vi "WriteToMeasArray.vi"(8 "error in (no error)":errorcluster, 10 "RoomAlert Device Reference":refnum<vi>, 11 "RoomAlert in":refnum<class "RoomAlert.lvclass">) -> (0 "error out":errorcluster, 3 "RoomAlert out":refnum<class "RoomAlert.lvclass">)   [LabVIEW 2018, in "SensorPlugins.lvlib" / "RoomAlert.lvclass"]
doc: "Updates to the measurement array all the values a user may measure from the RoomAlert."
uses:
  RoomAlert.lvclass
  TypeDefinitions/RoomAlertControls.ctl
panel:
  in  "Text Ring":u16(ring)
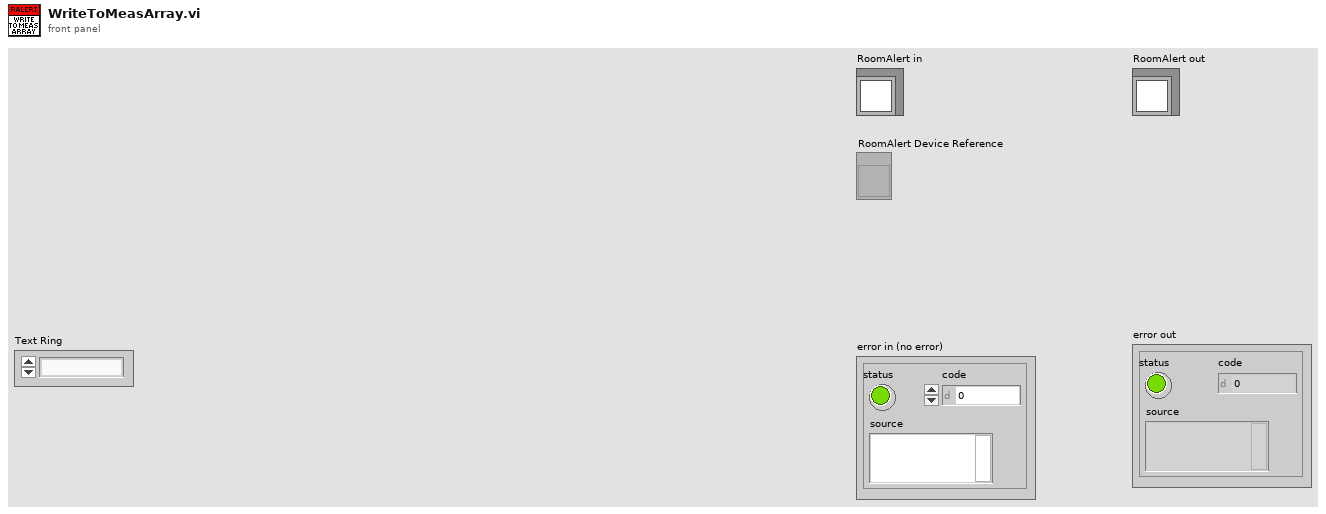
[diagram p1: front panel]
types:
  T1 = typedef "SensorPlugins.lvlib/RoomAlert.lvclass/RoomAlertControls.ctl" = cluster{"Connected?":bool, "IP Address of SNMP Device":string, "Port (161)":u16, "Community Name":string, "Measurements To Read Array":u16[], "Update LightTower?":bool, "LightTower":cluster{"Red":bool, "Amber":bool, "Green":bool, "Audio":bool}, "RoomAlert Model ID":string, "Sensor OID Numbers":string[][], "Sensor Light Tower OID Numbers":string[][]}[]
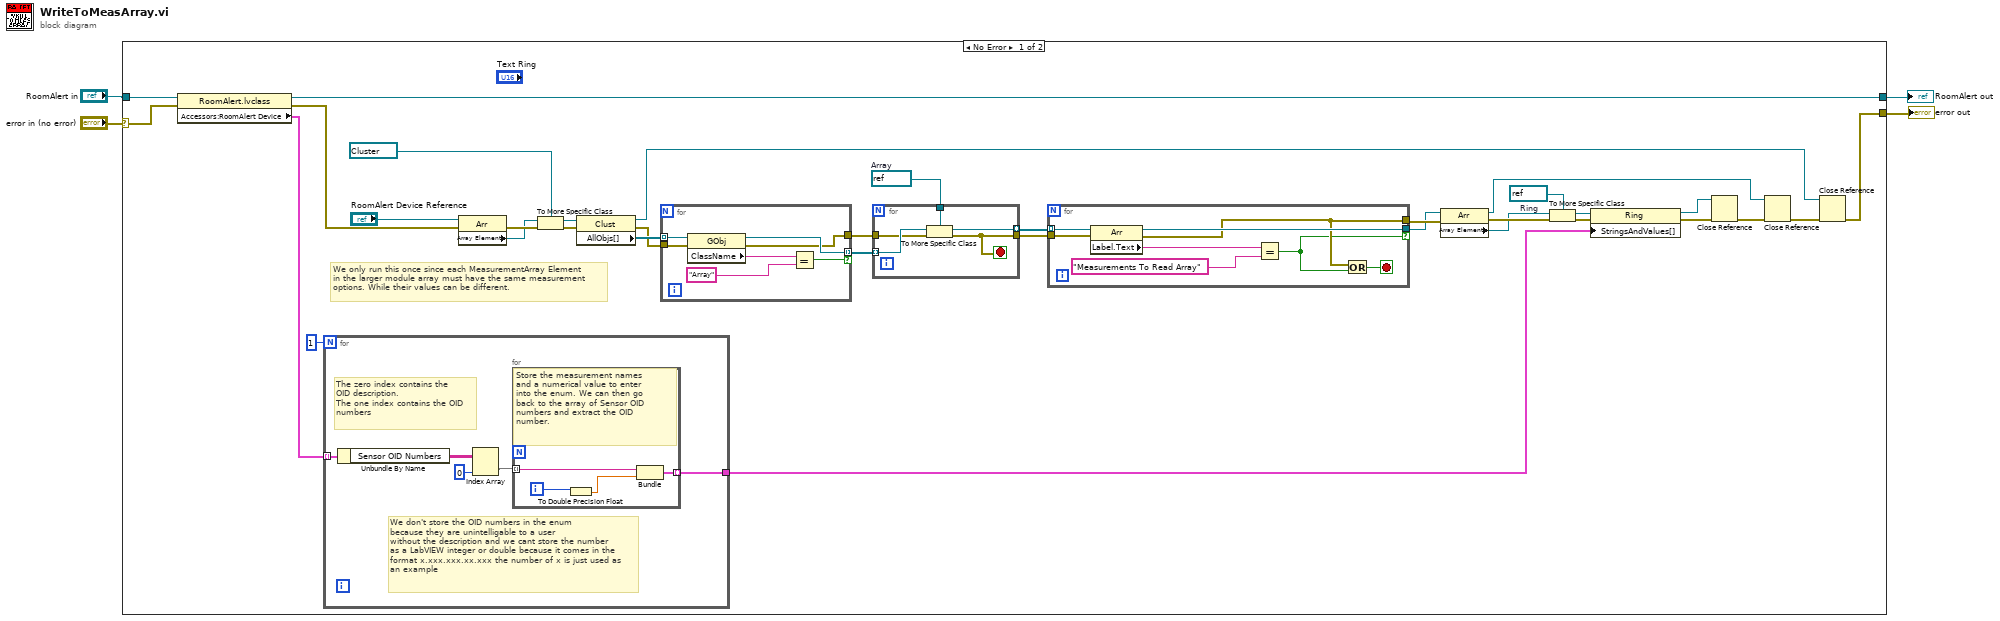
[diagram p0: block diagram]
diagram:
  n1 = case shown="No Error" "error in (no error)" {
    selector: "error in (no error)" -> [w37 w69]
    tunnel: [w20 w69] -> w1
    tunnel: [w36 w68] -> w2
    tunnel: "RoomAlert in" -> [w38 w68]
    frame No Error {
      w29 = refnum<vi> refnum  # Ring
      w10 = refnum<vi> refnum  # Array
      # "We only run this once since each MeasurementArray Element\nin the larger module array must have the same measurement \noptions. While their values can be different."
      n2 = property class="RoomAlert.lvclass"(reference=w38, error in=w37) -> (reference out=w36:refnum<class "RoomAlert.lvclass">, error out=w35:errorcluster, "Accessors:RoomAlert Device"=w6:T1)
      n3 = for {
        N: 1 -> [_]
        tunnel: w6 -> [w50] mode=indexing
        tunnel: [w49] -> w15
        # "We don't store the OID numbers in the enum\nbecause they are unintelligable to a user\nwithout the description and we cant store the number\nas a LabVIEW integer or double because it comes in the \nformat x.xxx.xxx.xx.xxx the number of x is just used as \nan example"
        # "The zero index contains the\nOID description.\nThe one index contains the OID\nnumbers"
        n4 = Unbundle By Name(w50) -> ("Sensor OID Numbers"=w48:string[][])
        n5 = Index Array(array=w48, index (col)=0 ("disabled index (col)")) -> (element=w46:string[])  [unwired: 1 in]
        n6 = for {
          tunnel: [w53] -> w49 mode=indexing
          tunnel: w46 -> [w52] mode=indexing
          i -> [w51]
          # "Store the measurement names \nand a numerical value to enter\ninto the enum. We can then go \nback to the array of Sensor OID\nnumbers and extract the OID \nnumber."
          n7 = To Double Precision Float(number=w51) -> (double precision float=w54:dbl)
          n8 = Bundle("String"=w52, w54) -> (w53:cluster{"String":string, dbl})  [unwired: 1 in]
        }
      }
      n9 = property class="Arr"(reference="RoomAlert Device Reference", error in=w35) -> (error out=w34:errorcluster, "Array Element"=w33:refnum<vi>)  [unwired: 1 out]
      n10 = To More Specific Class(target class=refnum<vi> refnum ("Text Ring"), reference=w33, error in=w34) -> (specific class reference=w30:refnum<vi>, error out=w31:errorcluster)
      n11 = property class="Clust"(reference=w30, error in=w31) -> (reference out=w17:refnum<vi>, error out=w13:errorcluster, "AllObjs[]"=w14:refnum<vi>[])
      n12 = for {
        tunnel: w14 -> [w45] mode=indexing
        tunnel: [w44] -> w11 mode=indexing if=w41
        tunnel: w13 -> [w42]
        tunnel: [w40] -> w12
        n13 = property class="GObj"(reference=w45, error in=w42) -> (reference out=w44:refnum<vi>, error out=w40:errorcluster, "ClassName"=w39:string)
        n14 = Equal?(x=w39, y="Array" ("ClassName")) -> (x = y?=w41:bool)
      }
      n15 = for {
        tunnel: w12 -> [w57]
        tunnel: w11 -> [w58] mode=indexing
        tunnel: w10 -> [w59]
        tunnel: [w56] -> w9 mode=indexing
        tunnel: [w55] -> w8
        stop <- w55 stop-if-true
        n16 = To More Specific Class(target class=w59, reference=w58, error in=w57) -> (specific class reference=w56:refnum<vi>, error out=w55:errorcluster)
      }
      n17 = for {
        tunnel: w9 -> [w67] mode=indexing
        tunnel: [w66] -> w16 if=w60
        tunnel: w8 -> [w64]
        tunnel: [w62] -> w18
        stop <- w63 stop-if-true
        n18 = property class="Arr"(reference=w67, error in=w64) -> (reference out=w66:refnum<vi>, error out=w62:errorcluster, "Label.Text"=w61:string)
        n19 = Equal?(x=w61, y="Measurements To Read Array" ("ClassName")) -> (x = y?=w60:bool)
        n20 = Or(x=w62, y=w60) -> (x .or. y?=w63:bool)
      }
      n21 = property class="Arr"(reference=w16, error in=w18) -> (reference out=w19:refnum<vi>, error out=w28:errorcluster, "Array Element"=w27:refnum<vi>)
      n22 = To More Specific Class(target class=w29, reference=w27, error in=w28) -> (specific class reference=w25:refnum<vi>, error out=w26:errorcluster)
      n23 = property class="Ring"(reference=w25, error in=w26, "StringsAndValues[]"=w15) -> (reference out=w23:refnum<vi>, error out=w24:errorcluster)
      n24 = Close Reference(reference=w23, error in (no error)=w24) -> (error out=w22:errorcluster)
      n25 = Close Reference(reference=w19, error in (no error)=w22) -> (error out=w21:errorcluster)
      n26 = Close Reference(reference=w17, error in (no error)=w21) -> (error out=w20:errorcluster)
    }
    frame Error {
    }
  }
  "error out" <- w1
  "RoomAlert out" <- w2
